vi "Final_Arm_Simulation.vi"(8 "Angle 2":dbl(knob)=-72.06882847083946 scale=-90.0..90.0, 9 "Angle1":dbl(knob)=-45.83837436417874 scale=-90.0..90.0, 10 "L 2":dbl(slide)=115.0 scale=0.0..200.0, 11 "L 1":dbl(slide)=80.0 scale=0.0..200.0) -> (1 "end effector":cluster{dbl, dbl}={159.01647214211073, 1.9100783062530127} {"?" format="%.1f"; "?" format="%#.1f"}, 3 "2D Picture":picture)   [LabVIEW 2024]
panel:
  out "angle":dbl
  out "mag":dbl
  # "A 2"
  # "L1"
  # "L2"
  # "A 1"
  # "mm"
  # "mm"
  # "mm"
  # "mm"
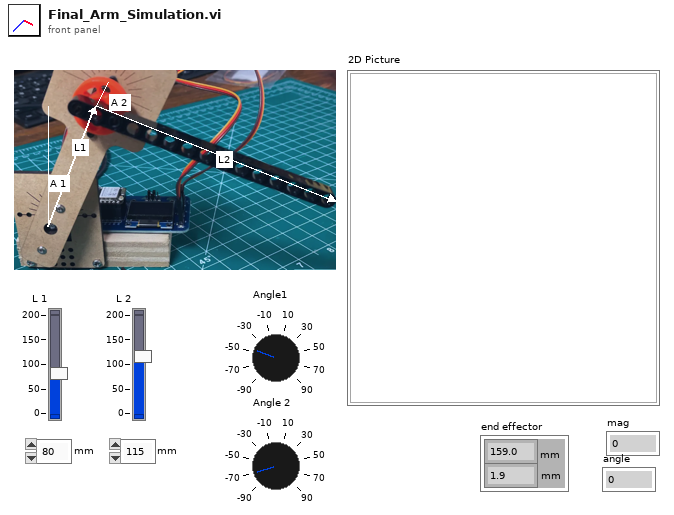
[diagram p1: front panel]
types:
  T1 = cluster{"Width":u16, "Style":enum32{"Solid", "Dash", "Dot", "DashDot", "DashDotDot"}}
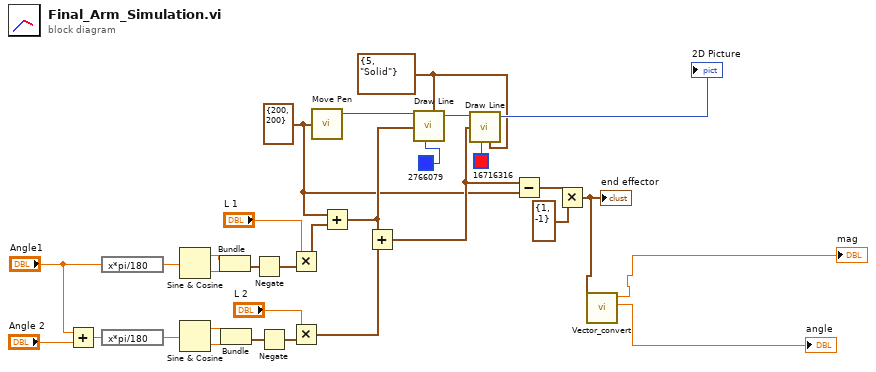
[diagram p0: block diagram]
diagram:
  w15 = T1 {"Width"=5, "Style"=enum."Solid"} ("pen")
  w4 = cluster{"x":i16, "y":i16} {"x"=200, "y"=200} ("new position")
  n1 = Add(x="Angle1", y="Angle 2") -> (x+y=w19:dbl)
  n2 = expression code="x*pi/180"("Angle1") -> (w30:dbl)
  n3 = expression code="x*pi/180"(w19) -> (w26:dbl)
  n4 = Sine & Cosine(0:w30) -> (1:w10:dbl, 2:w9:dbl)
  n5 = Sine & Cosine(0:w26) -> (1:w7:dbl, 2:w6:dbl)
  n6 = Bundle "Bundle"(w10, w9) -> (w29:cluster{dbl, dbl})  [unwired: 1 in]
  n7 = Bundle(w7, w6) -> (w27:cluster{dbl, dbl})  [unwired: 1 in]
  n8 = Negate(x=w29) -> (-x=w8:cluster{dbl, dbl})
  n9 = Negate(x=w27) -> (-x=w5:cluster{dbl, dbl})
  n10 = Multiply(x="L 1", y=w8) -> (x*y=w28:cluster{dbl, dbl})
  n11 = Multiply(x="L 2", y=w5) -> (x*y=w24:cluster{dbl, dbl})
  n12 = call <vilib>:"Move Pen.vi"("new position"=w4) -> ("new picture"=w31:picture)  [unwired: 4 in]
  n13 = Add(x=w4, y=w28) -> (x+y=w23:cluster{dbl, dbl})
  n14 = Add(x=w24, y=w23) -> (x+y=w14:cluster{dbl, dbl})
  n15 = call <vilib>:"Draw Line.vi"("picture"=w31, "end point"=w23, "color(black)"=u32 2766079, "pen"=w15) -> ("new picture"=w25:picture)  [unwired: 5 in]
  n16 = call <vilib>:"Draw Line.vi"("picture"=w25, "end point"=w14, "color(black)"=u32 16716316, "pen"=w15) -> ("new picture"=→"2D Picture":picture)  [unwired: 5 in]
  n17 = Subtract(x=w14, y=w4) -> (x-y=w13:cluster{dbl, dbl})
  n18 = Multiply(x=w13, y=cluster{"x":i16, "y":i16} {"x"=1, "y"=-1} ("new position")) -> (x*y=w1:cluster{dbl, dbl})
  "end effector" <- w1
  n19 = call <userlib>:"Vector_convert.vi"("x,y"=w1) -> ("angle"=→"angle":dbl, "mag"=→"mag":dbl)  [unwired: 9 in]
